vi "p1.vi"() -> ()   [LabVIEW 2021, in "d2.lvlib"]
uses:
  d2.lvlib
  AOC/AOC.lvlib
panel:
  in  "Example":string="A Y\nB X\nC Z"
  in  "Example":bool
  out "Answer":i64=10624
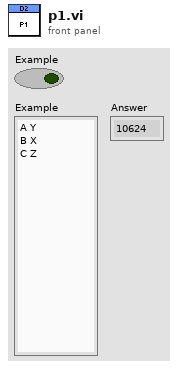
[diagram p1: front panel]
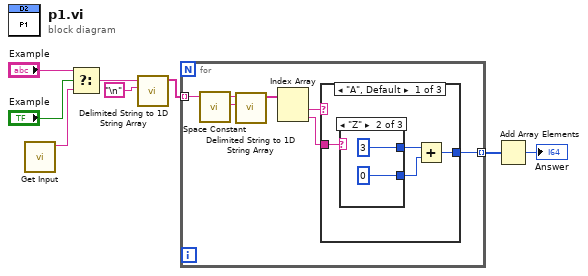
[diagram p0: block diagram]
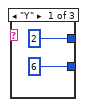
[diagram p2: hidden frame]
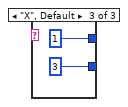
[diagram p3: hidden frame]
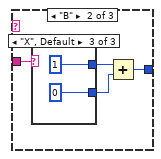
[diagram p4: hidden frame]
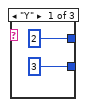
[diagram p5: hidden frame]
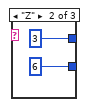
[diagram p6: hidden frame]
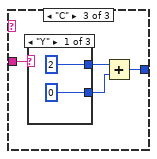
[diagram p7: hidden frame]
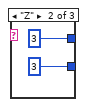
[diagram p8: hidden frame]
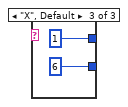
[diagram p9: hidden frame]
diagram:
  n1 = call "Get Input.vi"() -> ("Input"=w6:string)  [unwired: 11 in]
  n2 = Select(t="Example", s="Example", f=w6) -> (s? t:f=w5:string)
  n3 = call <vilib>:"Delimited String to 1D String Array.vi"("delimiter"="\n", "delimited string"=w5) -> ("string array"=w3:string[])  [unwired: 9 in]
  n4 = for {
    tunnel: w3 -> [w9] mode=indexing
    tunnel: [w12] -> w8 mode=indexing
    n5 = call <vilib>:"Space Constant.vi"() -> ("String"=w11:string)
    n6 = call <vilib>:"Delimited String to 1D String Array.vi"("delimiter"=w11, "delimited string"=w9) -> ("string array"=w10:string[])  [unwired: 9 in]
    n7 = Index Array(array=w10) -> (element #1=w14:string, element #2=w13:string)  [unwired: 2 in]
    n8 = case shown="\"A\", Default" w14 {
      tunnel: w13 -> [w18 w28 w38]
      tunnel: [w15 w25 w35] -> w12
      frame "A", Default {
        n9 = case shown="\"Z\"" w18 {
          tunnel: [6 0 3] -> w16
          tunnel: [2 3 1] -> w17
          frame "Y" {
          }
          frame "Z" {
          }
          frame "X", Default {
          }
        }
        n10 = Add(x=w17, y=w16) -> (x+y=w15:i32)
      }
      frame "B" {
        n11 = case shown="\"X\", Default" w28 {
          tunnel: [3 6 0] -> w26
          tunnel: [2 3 1] -> w27
          frame "Y" {
          }
          frame "Z" {
          }
          frame "X", Default {
          }
        }
        n12 = Add(x=w27, y=w26) -> (x+y=w25:i32)
      }
      frame "C" {
        n13 = case shown="\"Y\"" w38 {
          tunnel: [0 3 6] -> w36
          tunnel: [2 3 1] -> w37
          frame "Y" {
          }
          frame "Z" {
          }
          frame "X", Default {
          }
        }
        n14 = Add(x=w37, y=w36) -> (x+y=w35:i32)
      }
    }
  }
  n15 = Add Array Elements(numeric array=w8) -> (sum=→"Answer":i32)
